vi "Configure AC Current.vi"(0 "VISA resource name":refnum<visa-resource-name>, 1 "Aperture Seconds":dbl, 2 "Bandwidth (30)":u16(ring) items=["3", "30", "300"], 5 "Auto Range? (T: Auto)":bool, 7 "Manual Range":dbl=3.0, 9 "Set Aperture or NPLC":bool=TRUE, 11 "error in (no error)":errorcluster, 12 "NPLC":dbl=1.0) -> (4 "VISA resource name out":refnum<visa-resource-name>, 15 "error out":errorcluster)   [LabVIEW 2021, in "Keithley DMM7510.lvlib"]
doc: "This VI configures the AC Current measurement and the related parameters."
uses:
  Keithley DMM7510.lvlib
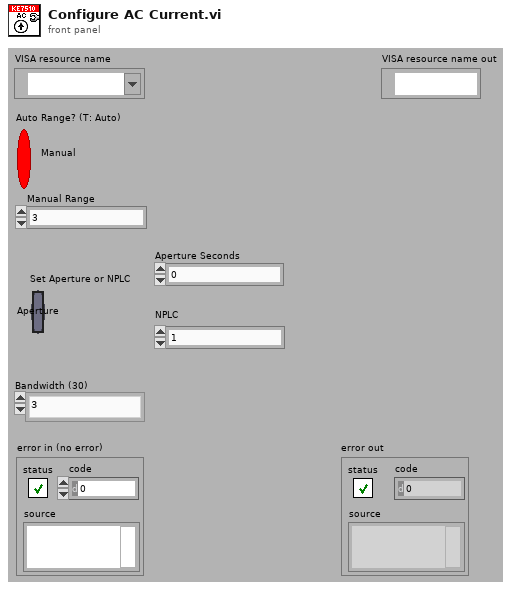
[diagram p1: front panel]
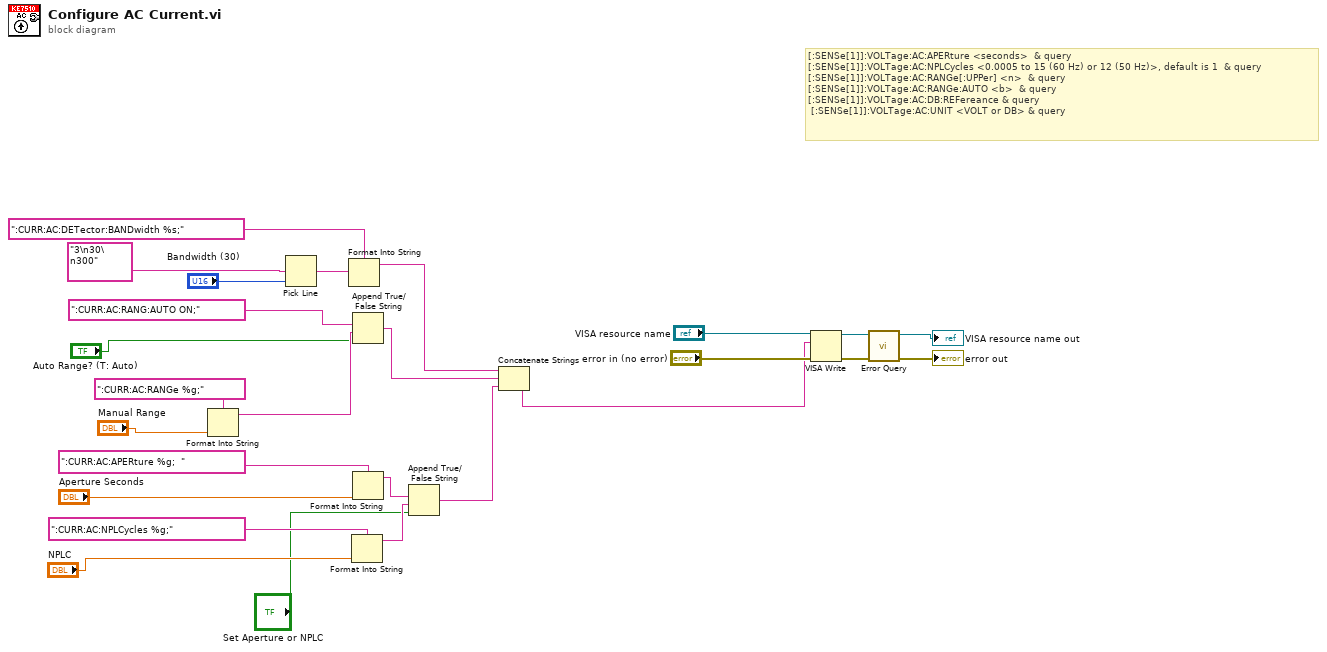
[diagram p0: block diagram]
diagram:
  # "[:SENSe[1]]:VOLTage:AC:APERture <seconds>  & query\n[:SENSe[1]]:VOLTage:AC:NPLCycles <0.0005 to 15 (60 Hz) or 12 (50 Hz)>, default is 1  & query\n[:SENSe[1]]:VOLTage:AC:RANGe[:UPPer] <n>  & query\n[:SENSe[1]]:VOLTage:AC:RANGe:AUTO <b>  & query\n[:SENSe[1]]:VOLTage:AC:DB:REFereance & query\n [:SENSe[1]]:VOLTage:AC:UNIT <VOLT or DB> & query"
  n1 = Format Into String(format string=":CURR:AC:RANGe %g;", "Manual Range") -> (resulting string=w21:string)  [unwired: 2 in, 1 out]
  n2 = Pick Line(multi-line string="3\n30\n300", line index="Bandwidth (30)") -> (output string=w10:string)  [unwired: 1 in]
  n3 = Format Into String(format string=":CURR:AC:DETector:BANDwidth %s;", w10) -> (resulting string=w18:string)  [unwired: 2 in, 1 out]
  n4 = Format Into String(format string=":CURR:AC:NPLCycles %g;", "NPLC") -> (resulting string=w3:string)  [unwired: 2 in, 1 out]
  n5 = Append True/False String(1:"Auto Range? (T: Auto)", 2:w21, 3:":CURR:AC:RANG:AUTO ON;") -> (0:w17:string)  [unwired: 1 in]
  n6 = Format Into String(format string=":CURR:AC:APERture %g;  ", "Aperture Seconds") -> (resulting string=w4:string)  [unwired: 2 in, 1 out]
  n7 = Append True/False String(1:"Set Aperture or NPLC", 2:w3, 3:w4) -> (0:w1:string)  [unwired: 1 in]
  n8 = Concatenate Strings(w18, w17, w1) -> (w16:string)
  n9 = VISA Write(VISA resource name="VISA resource name", write buffer=w16, error in (no error)="error in (no error)") -> (VISA resource name out=w15:refnum<visa-resource-name>, error out=w14:errorcluster)  [unwired: 1 out]
  n10 = call "Error Query.vi"("error in (no error)"=w14, "VISA resource name"=w15) -> ("error out"=→"error out":errorcluster, "VISA resource name out"=→"VISA resource name out":refnum<visa-resource-name>)  [unwired: 6 in, 2 out]
